vi "Math Compute Segment Intersection with Unit Circle.vi"(8 "Error In":errorcluster, 10 "Point 2":cluster{"X":dbl, "Y":dbl}, 11 "Point 1":cluster{"X":dbl, "Y":dbl}) -> (0 "Error Out":errorcluster, 2 "Intersection 2":cluster{"x1m":dbl, "y1m":dbl}, 3 "Intersection 1":cluster{"x1p":dbl, "y1p":dbl})   [LabVIEW 2021, in "Math.lvlib"]
uses:
  Math.lvlib
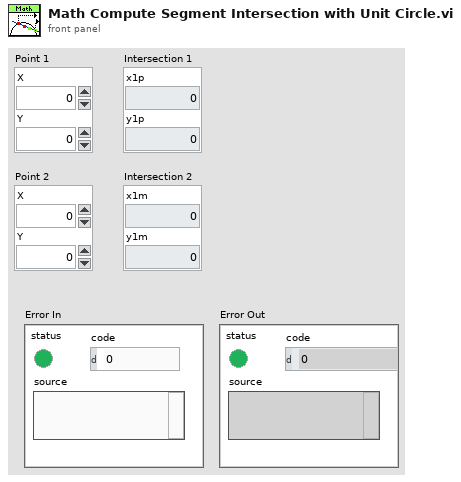
[diagram p1: front panel]
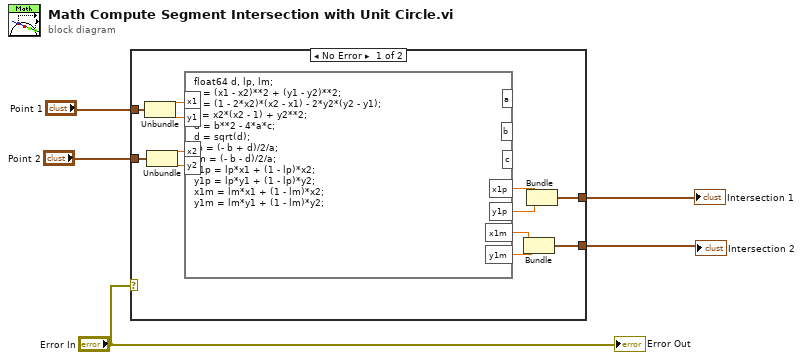
[diagram p0: block diagram]
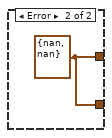
[diagram p2: hidden frame]
diagram:
  n1 = case shown="No Error" "Error In" {
    tunnel: "Point 2" -> [w15 _]
    tunnel: "Point 1" -> [w12 _]
    tunnel: [w11 w18] -> w3
    tunnel: [w8 w18] -> w2
    frame No Error {
      n2 = Unbundle(w12) -> ("X"=w14:dbl, "Y"=w13:dbl)
      n3 = Unbundle(w15) -> ("X"=w16:dbl, "Y"=w17:dbl)
      n4 = formula code="float64 d, lp, lm;\na = (x1 - x2)**2 + (y1 - y2)**2;\nb = (1 - 2*x2)*(x2 - x1) - 2*y2*(y2 - y1);\nc = x2*(x2 - 1) + y2**2;\nd = b**2 - 4*a*c;\nd = sqrt(d);\nlp = (- b + d)/2/a;\nlm = (- b - d)/2/a;\nx1p = lp*x1 + (1 - lp)*x2;\ny1p = lp*y1 + (1 - lp)*y2;\nx1m = lm*x1 + (1 - lm)*x2;\ny1m = lm*y1 + (1 - lm)*y2;"("x1"=w14, "y1"=w13, "x2"=w16, "y2"=w17) -> ("x1p"=w6:dbl, "x1m"=w9:dbl, "y1p"=w7:dbl, "y1m"=w10:dbl)  [unwired: 3 out]
      n5 = Bundle("x1m"=w9, "y1m"=w10) -> (w11:cluster{"x1m":dbl, "y1m":dbl})  [unwired: 1 in]
      n6 = Bundle("x1p"=w6, "y1p"=w7) -> (w8:cluster{"x1p":dbl, "y1p":dbl})  [unwired: 1 in]
    }
    frame Error {
      w18 = cluster{"x1p":dbl, "y1p":dbl} {"x1p"=nan, "y1p"=nan}
    }
  }
  "Intersection 2" <- w3
  "Intersection 1" <- w2
  "Error Out" <- "Error In"
